vi "FixCodeSpacing.vi"(11 "Code":string) -> (3 "Cleaned for SPIKE":string)   [LabVIEW 2020]
panel:
  out "Array 2":i32[](array[numeric])
  out "Array":i32[](array[numeric])
  out "Indents":i32[](array[numeric])
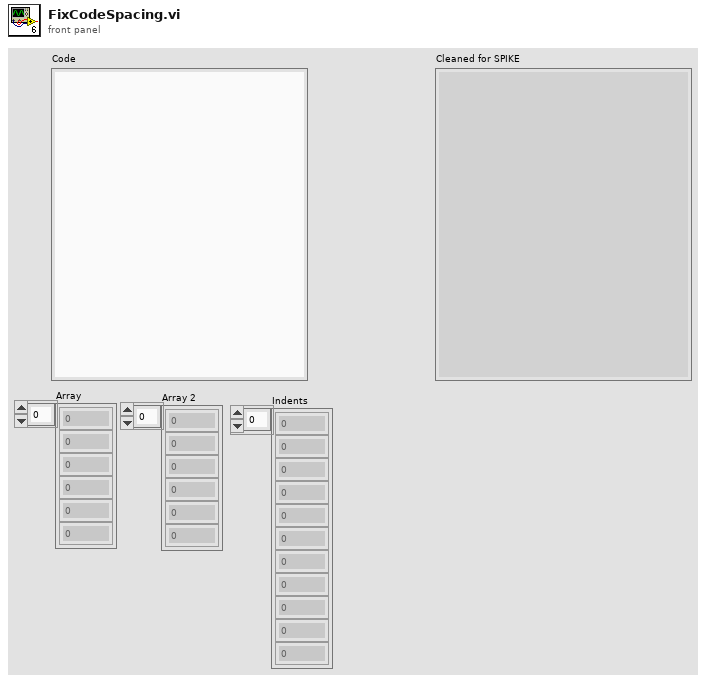
[diagram p1: front panel]
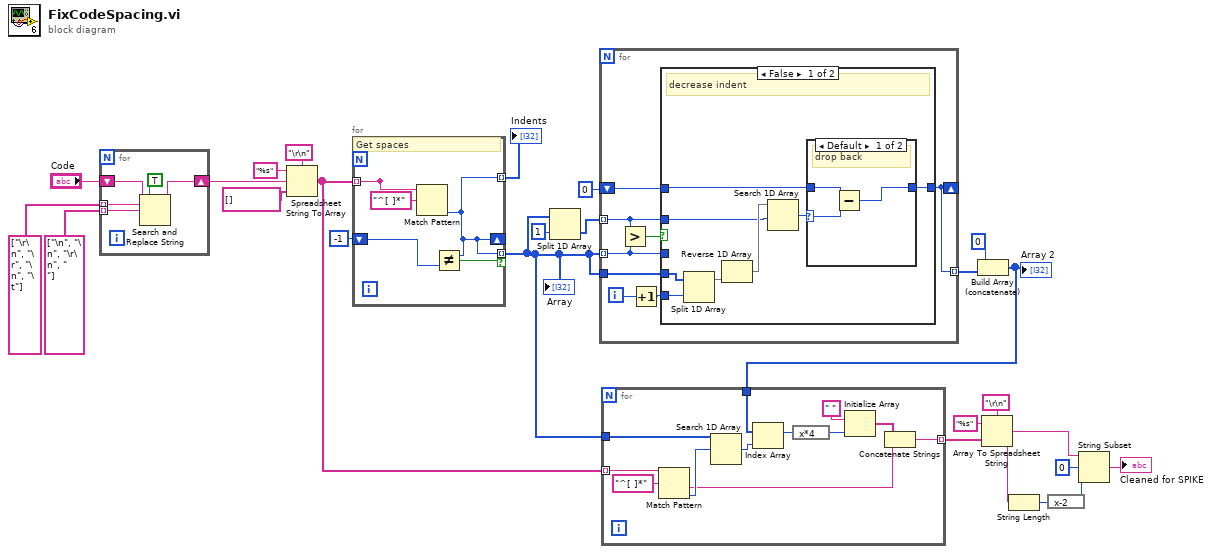
[diagram p0: block diagram]
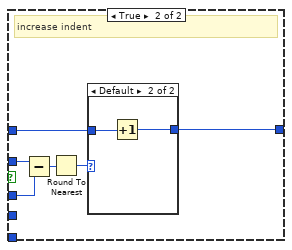
[diagram p3: hidden frame]
diagram:
  n1 = for {
    tunnel: string[] ["\r\n", "\r", "\n", "\t"] -> [w28] mode=indexing
    tunnel: string[] ["\n", "\n", "\r\n", "    "] -> [w27] mode=indexing
    shift-right: [w26] -> w18
    shift-left: "Code" -> [w30]
    n2 = Search and Replace String(replace all?=TRUE ("replace all? (F)"), input string=w30, search string=w28, replace string=w27) -> (result string=w26:string)  [unwired: 4 in, 3 out]
  }
  n3 = Spreadsheet String To Array(delimiter (Tab)="\r\n" ("replace string (\"\")"), format string="%s", spreadsheet string=w18, array type (2D Dbl)=string[] []) -> (array=w12:string[])
  n4 = for {
    tunnel: [w35] -> _ mode=indexing
    tunnel: w12 -> [w35] mode=indexing
    tunnel: [w32] -> w19 mode=indexing
    shift-right: [w32] -> _
    shift-left: -1 ("offset past match") -> [w33]
    tunnel: [w32] -> w13 mode=indexing if=w31
    # "Get spaces"
    n5 = Match Pattern(string=w35, regular expression="^[ ]*") -> (offset past match=w32:i32)  [unwired: 1 in, 3 out]
    n6 = Not Equal?(x=w32, y=w33) -> (x != y?=w31:bool)
  }
  "Indents" <- w19
  "Array" <- w13
  n7 = Split 1D Array(array=w13, index=1) -> (second subarray=w15:i32[])  [unwired: 1 out]
  n8 = for {
    tunnel: w13 -> [w37] mode=indexing
    tunnel: w15 -> [w41] mode=indexing
    shift-right: [w36] -> _
    shift-left: 0 ("n") -> [w42]
    tunnel: w13 -> [w40]
    tunnel: [w36] -> w8 mode=indexing
    i -> [w39]
    n9 = Greater?(x=w41, y=w37) -> (0:w43:bool)
    n10 = Increment(x=w39) -> (x+1=w38:i32)
    n11 = case shown="False" w43 {
      tunnel: w42 -> [w50 w60]
      tunnel: [w49 w61] -> w36
      tunnel: w41 -> [w47 w57]
      tunnel: w40 -> [w46 _]
      tunnel: w38 -> [w44 _]
      tunnel: w37 -> [_ w56]
      frame False {
        # "decrease indent"
        n12 = Split 1D Array(array=w46, index=w44) -> (first subarray=w45:i32[])  [unwired: 1 out]
        n13 = Reverse 1D Array(array=w45) -> (reversed array=w48:i32[])
        n14 = Search 1D Array(1D array=w48, element=w47) -> (index of element=w51:i32)  [unwired: 1 in]
        n15 = case shown="Default" w51 {
          selector: w51 -> [w53 _]
          tunnel: w50 -> [w54 w55]
          tunnel: [w52 w55] -> w49
          frame Default {
            # "drop back"
            n16 = Subtract(x=w54, y=w53) -> (x-y=w52:i32)
          }
          frame -1 {
            # "not aligned"
          }
        }
      }
      frame True {
        # "increase indent"
        n17 = Subtract(x=w57, y=w56) -> (x-y=w58:i32)
        n18 = Round To Nearest(number=w58) -> (nearest integer value=w59:i32)
        n19 = case shown="Default" w59 {
          tunnel: w60 -> [w62 w64]
          tunnel: [w62 w63] -> w61
          frame 0, 1 {
          }
          frame Default {
            n20 = Increment(x=w64) -> (x+1=w63:i32)
          }
        }
      }
    }
  }
  n21 = Build Array (concatenate)(0 ("n"), w8) -> (w6:i32[])
  "Array 2" <- w6
  n22 = for {
    tunnel: w13 -> [w74]
    tunnel: w12 -> [w75] mode=indexing
    tunnel: [w68] -> w11 mode=indexing
    tunnel: w6 -> [w66]
    n23 = Match Pattern(string=w75, regular expression="^[ ]*") -> (after substring=w69:string, offset past match=w73:i32)  [unwired: 1 in, 2 out]
    n24 = Search 1D Array(1D array=w74, element=w73) -> (index of element=w72:i32)  [unwired: 1 in]
    n25 = Index Array(array=w66, index=w72) -> (element=w65:i32)
    n26 = expression code="x*4"(w65) -> (w67:i32)
    n27 = Initialize Array(" " ("regular expression"), w67) -> (w70:string[])
    n28 = Concatenate Strings(w70, w69) -> (w68:string)
  }
  n29 = Array To Spreadsheet String(delimiter (Tab)="\r\n" ("replace string (\"\")"), array=w11, 3:"%s" ("format string")) -> (spreadsheet string=w3:string)
  n30 = String Length(string=w3) -> (length=w2:i32)
  n31 = expression code="x-2"(w2) -> (w1:i32)
  n32 = String Subset(string=w3, offset (0)=0, length (rest)=w1) -> (substring=→"Cleaned for SPIKE":string)
